vi "test_Path (programfiles).vi"(8 "error in (no error)":errorcluster, 11 "TestCase in":refnum<class "Read Section - Path Tests.lvclass">) -> (0 "error out":errorcluster, 3 "TestCase out":refnum<class "Read Section - Path Tests.lvclass">)   [LabVIEW 2017, in "Read Section - Path Tests.lvclass"]
uses:
  Read Section - Path Tests.lvclass
  C:/Development/Reuse-libraries/File IO/_Unit Test/Read File Tests/Read File Tests.lvclass
  <vilib>/Utility/sysdir.llb/System Directory Type.ctl
  Read File Tests.lvclass/Read File Tests.ctl
  Read/Read Section - Path.vi
  <vilib>/addons/_JKI Toolkits/VI Tester/TestCase.llb/TestCase.lvclass
  TSC File IO.lvlib
  Read File Tests.lvclass
  C:/Program Files (x86)/National Instruments/LabVIEW 2017/vi.lib/addons/_JKI Toolkits/VI Tester/TestCase.llb/TestCase.lvclass
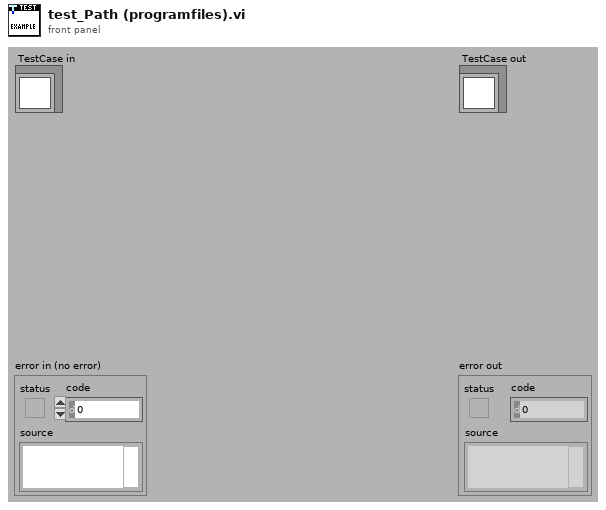
[diagram p1: front panel]
types:
  T1 = typedef "System Directory Type.ctl" = i32
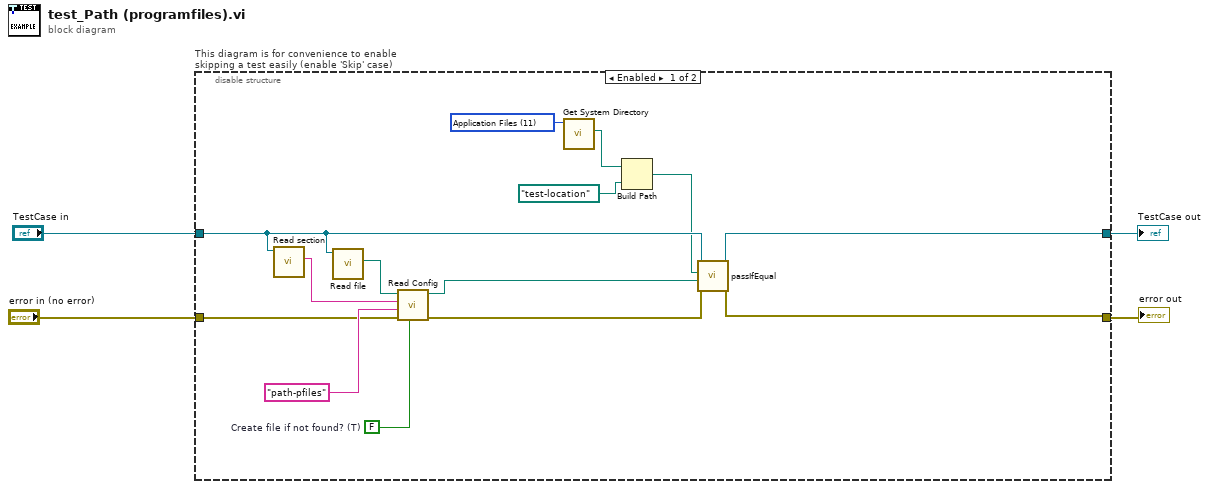
[diagram p0: block diagram]
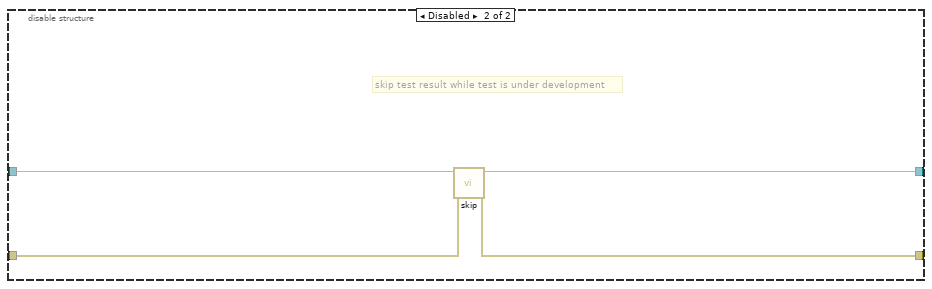
[diagram p2: hidden frame]
diagram:
  n1 = disable-structure "This diagram is for convenience to enable skipping a test easily (enable 'Skip' case)" shown="Enabled" {
    disable-tunnel: "TestCase in" -> [w11 w22]
    disable-tunnel: [w18 w20] -> w1
    disable-tunnel: [w17 w21] -> w3
    disable-tunnel: "error in (no error)" -> [w14 w19]
    frame Enabled {
      w7 = T1 11 items=["User Home"=0, "User Desktop"=1, "User Documents"=2, "User Application Data"=3, "User Preferences"=4, "User Temporary"=5, "Public Documents"=6, "Public Application Data"=7, "Public Preferences"=8, "Public Cache"=13, "System Core Libraries"=9, "System Installed Libraries"=10, "Application Files"=11, "Boot Volume Root"=12] ("system directory type")
      w15 = FALSE  # Create file if not found? (T)
      n2 = call "Read section.vi"("Read File Tests in"=w11) -> ("section"=w10:string)  [unwired: 8 in, 2 out]
      n3 = call "Read file.vi"("Read File Tests in"=w11) -> ("file"=w12:path)  [unwired: 8 in, 2 out]
      n4 = call-poly "Read Config.vi"("Create file if not found? (T)"=w15, "error in (no error)"=w14, "key"="path-pfiles", "section"=w10, "Path"=w12) -> ("error out"=w13:errorcluster, "value"=w9:path)  [unwired: 5 in]
      n5 = call <vilib>:"Get System Directory.vi"("system directory type"=w7) -> ("system directory"=w6:path)  [unwired: 10 in]
      n6 = Build Path(base path=w6, name or relative path=path "test-location") -> (appended path=w5:path)
      n7 = call-dynamic "passIfEqual.vi"("error in (no error)"=w13, "y"=w9, "x"=w5, "TestCase in"=w11) -> ("error out"=w17:errorcluster, "TestCase out"=w18:refnum<class "Read Section - Path Tests.lvclass">)  [unwired: 6 in]
    }
    frame Disabled {
      # "skip test result while test is under development"
      n8 = call <vilib>:"skip.vi"("error in (no error)"=w19, "TestCase in"=w22) -> ("error out"=w21:errorcluster, "TestCase out"=w20:refnum<class "Read Section - Path Tests.lvclass">)  [unwired: 8 in]
    }
  }
  "error out" <- w3
  "TestCase out" <- w1
